vi "Global Excitation Current.vi"() -> ()   [LabVIEW 2019]
panel:
  in  "Excitation Current":dbl
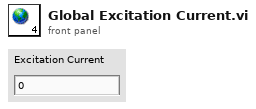
[diagram p1: front panel]
diagram:
